vi "Add Timing Channels.vi"(8 "error in":errorcluster, 11 "custom device ref":T1 format="%.0x") -> (0 "error out":errorcluster, 3 "custom device ref out":T1 format="%.0x")   [LabVIEW 2020, in "Ballard ARINC 429 Scripting.lvlib"]
doc: "Adds 'Status' section and required channels including error status channels and asynchronous loop time."
uses:
  <vilib>/NI VeriStand/Custom Device API/Custom Device Item Ref.ctl
  Ballard ARINC 429 Scripting.lvlib
  <vilib>/NI VeriStand/Custom Device API/Custom Device API.lvlib
  Constants.vi
  <vilib>/NI VeriStand/Custom Device API/Custom Device Channel Type.ctl
  <vilib>/NI VeriStand/Custom Device API/Custom Device Channel.ctl
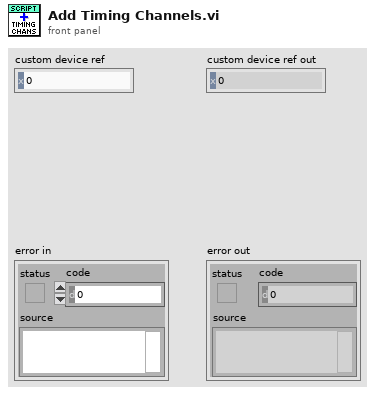
[diagram p1: front panel]
types:
  T1 = typedef "Custom Device API.lvlib/Custom Device Item Ref.ctl" = u64
  T2 = typedef "Custom Device API.lvlib/Custom Device Channel.ctl" = cluster{"Type":T3, "Units":string, "Default Value":dbl, "Faultable":bool, "Scalable":bool}
  T3 = typedef "Custom Device API.lvlib/Custom Device Channel Type.ctl" = enum16{"Input", "Output"}
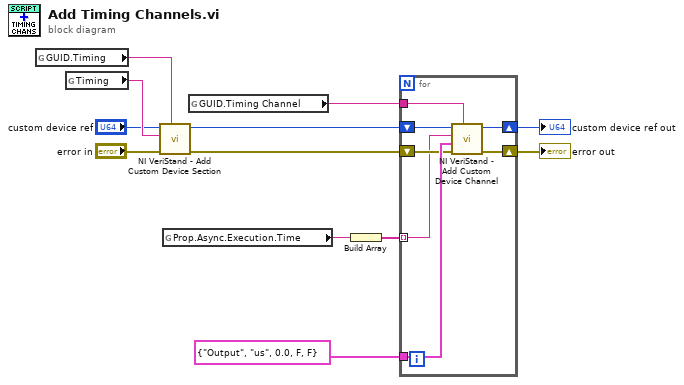
[diagram p0: block diagram]
diagram:
  n1 = global read "Constants.vi" "GUID.Timing"() -> (w11:string)
  n2 = global read "Constants.vi" "Timing"() -> (w12:string)
  n3 = call <vilib>:"NI VeriStand - Add Custom Device Section.vi"("GUID (Default Section)"=w11, "error in (no error)"="error in", "Section Name"=w12, "Parent Ref in"="custom device ref") -> ("error out"=w4:errorcluster, "Parent Ref out"=w5:T1)  [unwired: 4 in, 2 out]
  n4 = global read "Constants.vi" "Prop.Async.Execution.Time"() -> (w1:string)
  n5 = global read "Constants.vi" "GUID.Timing Channel"() -> (w8:string)
  n6 = Build Array(w1) -> (w6:string[])
  n7 = for {
    tunnel: w8 -> [w18]
    tunnel: T2 {"Type"=enum."Output", "Units"="us", "Default Value"=0.0, "Faultable"=FALSE, "Scalable"=FALSE} ("Channel") -> [w17]
    shift-right: [w14] -> w2
    shift-left: w5 -> [w19]
    shift-right: [w15] -> w3
    shift-left: w4 -> [w16]
    tunnel: w6 -> [w13] mode=indexing
    n8 = call <vilib>:"NI VeriStand - Add Custom Device Channel.vi"("GUID (Default Channel)"=w18, "error in (no error)"=w16, "Channel"=w17, "Channel Name"=w13, "Parent Ref in"=w19) -> ("error out"=w15:errorcluster, "Parent Ref out"=w14:T1)  [unwired: 3 in, 2 out]
  }
  "custom device ref out" <- w2
  "error out" <- w3
